vi "Quick Usb Find Modules.vi"(8 "error in (no error)":errorcluster, 10 "length":u32, 11 "nameList":string) -> (0 "error out":errorcluster, 2 "function return":i32, 3 "nameList out":string)   [LabVIEW 2011, in "QuickUSB.lvlib"]
doc: "QUSBLIB QRETURN QuickUsbFindModules(\n PQCHAR nameList,\n QULONG length);"
uses:
  QuickUSB.lvlib
  QuickUSB.dll
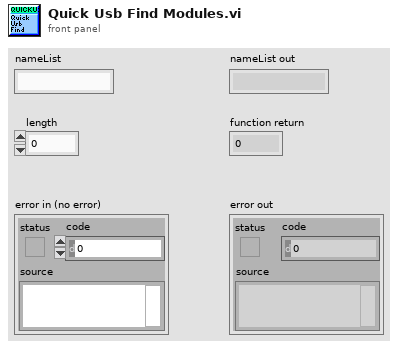
[diagram p1: front panel]
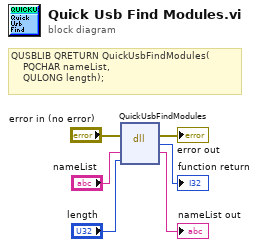
[diagram p0: block diagram]
diagram:
  # "QUSBLIB QRETURN QuickUsbFindModules(\n    PQCHAR nameList,\n    QULONG length);"
  n1 = dll-call lib="C:/QuickUSB/QuickUSB.*" fn="QuickUsbFindModules"(error in="error in (no error)", "nameList"="nameList", "length"="length") -> (error out=→"error out":errorcluster, →"function return":i32, "nameList"=→"nameList out":string)  [unwired: 3 in, 1 out]
